vi "Get GUI refs.vi"(8 "error in (no error)":errorcluster, 11 "DAQMH121119OrcaFlash in":refnum<class "DAQOrcaFlash.lvclass">) -> (0 "error out":errorcluster, 2 "Array":refnum<vi>[](array[refnum]), 3 "DAQMH121119OrcaFlash out":refnum<class "DAQOrcaFlash.lvclass">)   [LabVIEW 2012, in "DAQOrcaFlash.lvclass"]
uses:
  DAQOrcaFlash.lvclass
  DAQOrcaFlash.lvclass/DAQOrcaFlash.ctl
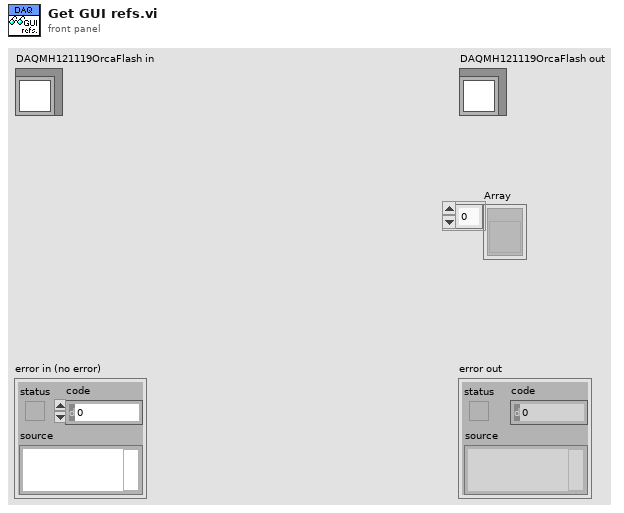
[diagram p1: front panel]
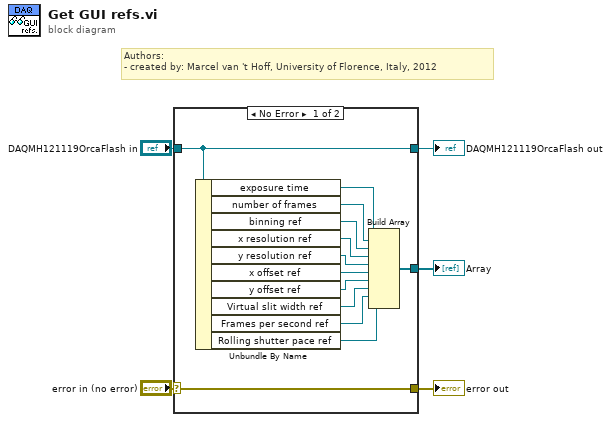
[diagram p0: block diagram]
diagram:
  # "Authors: \n- created by: Marcel van 't Hoff, University of Florence, Italy, 2012"
  n1 = case shown="No Error" "error in (no error)" {
    selector: "error in (no error)" -> [w18 w20]
    tunnel: [w18 w20] -> w4
    tunnel: [w17 w19] -> w2
    tunnel: "DAQMH121119OrcaFlash in" -> [w17 w19]
    tunnel: [w9 _] -> w1
    frame No Error {
      n2 = Unbundle By Name(w17) -> ("exposure time"=w16:refnum<vi>, "number of frames"=w15:refnum<vi>, "binning ref"=w14:refnum<vi>, "x resolution ref"=w13:refnum<vi>, "y resolution ref"=w12:refnum<vi>, "x offset ref"=w11:refnum<vi>, "y offset ref"=w10:refnum<vi>, "Virtual slit width ref"=w8:refnum<vi>, "Frames per second ref"=w6:refnum<vi>, "Rolling shutter pace ref"=w7:refnum<vi>)
      n3 = Build Array(w16, w15, w14, w13, w12, w11, w10, w8, w6, w7) -> (w9:refnum<vi>[])
    }
    frame Error {
    }
  }
  "error out" <- w4
  "DAQMH121119OrcaFlash out" <- w2
  "Array" <- w1
